vi "Stop.vi"(6 "Teller":refnum<class "Teller.lvclass">, 8 "Error in":errorcluster, 11 "TEMPLATE Actor in":refnum<class "TEMPLATE Actor.lvclass">) -> (0 "Error out":errorcluster, 3 "TEMPLATE Actor out":refnum<class "TEMPLATE Actor.lvclass">)   [LabVIEW 2020, in "_Template.lvlib" / "Templates.lvlib" / "TEMPLATE jettl Actor.lvlib" / "TEMPLATE Actor.lvlib" / "TEMPLATE Actor.lvclass"]
uses:
  jettl/jettl/Teller/Teller.lvclass
  TEMPLATE Actor.lvclass
  TEMPLATE Actor.lvclass/TEMPLATE Actor.ctl
  jettl/jettl/Stop jettl Msg/Stop/Stop.lvlib
  jettl/jettl/Stop jettl Msg/Stop/Recurse.vi
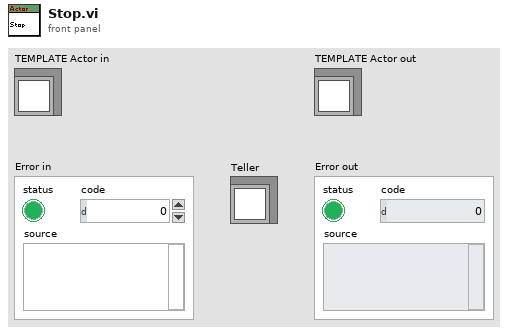
[diagram p1: front panel]
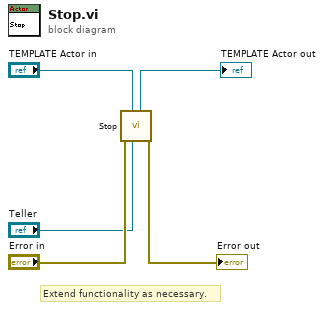
[diagram p0: block diagram]
diagram:
  # "Extend functionality as necessary."
  n1 = call-poly "Stop.vi"("Teller"="Teller", "Actor in"="TEMPLATE Actor in", "Error in"="Error in") -> ("Error out"=→"Error out":errorcluster, "Actor out"=→"TEMPLATE Actor out":refnum<class "TEMPLATE Actor.lvclass">)  [unwired: 7 in]
